vi "io_set_VISA_timeout.vi"(8 "error in":errorcluster caption="error in (no error)", 10 "VISA Timeout":u32=5000, 11 "VISA resource name":refnum<visa-resource-name>) -> (0 "error out":errorcluster, 2 "Old VISA Timeout":u32, 3 "VISA resource name out":refnum<visa-resource-name>)   [LabVIEW 2022 SP3, in "hmp4000_rsidr_core.lvlib"]
uses:
  hmp4000_rsidr_core.lvlib
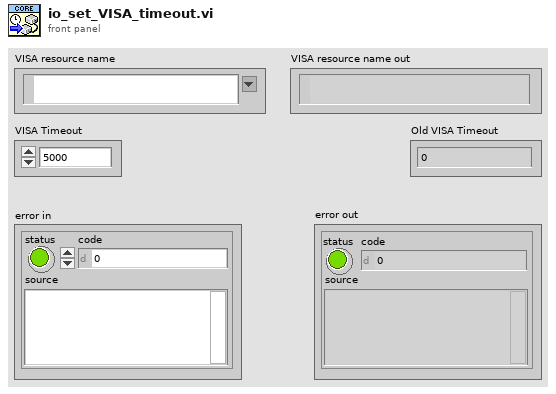
[diagram p1: front panel]
types:
  T1 = typedef "hmp4000_rsidr_core.lvlib/type_Session_Data.ctl" = cluster{"IDN string":string, "Instrument FW":string, "Instr type":string, "Instr type for err. msg.":string, "Installed Options":string[], "Ignore Error Messages":string, "Logging params":variant, "OPC Timeout":i32, "VISA Timeout":i32, "STB Poll VISA Timeout":i32, "Additional Flags":i32, "Wait Before Read":i32, "Wait Before Write":i32, "Option String Flags":i32, "IO Segment Size":i64, "VISA Access Mode":T2, "Interface Type":T3, "OPC Wait Mode":T4, "Bin Float Number  Format":T5, "Bin Integer Number Format":T6, "Simulate":bool, "VXIcapable":bool, "Duplicate Session":bool, "Add LF to Write":bool, "Logging":bool, "Fast Sweep":bool, "Query Instrument Status":bool, "Check Range":bool, "Check Options":bool}
  T2 = typedef "hmp4000_rsidr_core.lvlib/type_VisaAccessMode.ctl" = u16
  T3 = typedef "hmp4000_rsidr_core.lvlib/type_InterfaceType.ctl" = enum16{"Unknown", "GPIB", "VXI", "GPIB_VXI", "ASRL", "PXI", "TCPIP", "USB", "SOCKET"}
  T4 = typedef "hmp4000_rsidr_core.lvlib/type_OPC_Wait_Mode.ctl" = enum16{"STBpolling", "STBpollingSlow", "STBpollingSuperSlow", "ServiceRequest", "OPCquery"}
  T5 = typedef "hmp4000_rsidr_core.lvlib/type_Binary_Float_Number_Format.ctl" = enum16{"Float_4_Bytes_Swapped", "Float_4_Bytes", "Double_8_Bytes_Swapped", "Double_8_Bytes"}
  T6 = typedef "hmp4000_rsidr_core.lvlib/type_Binary_Integer_Number_Format.ctl" = enum16{"Int32_4_Bytes_Swapped", "Int32_4 Bytes", "Int16_2_Bytes_Swapped", "Int16_2_Bytes"}
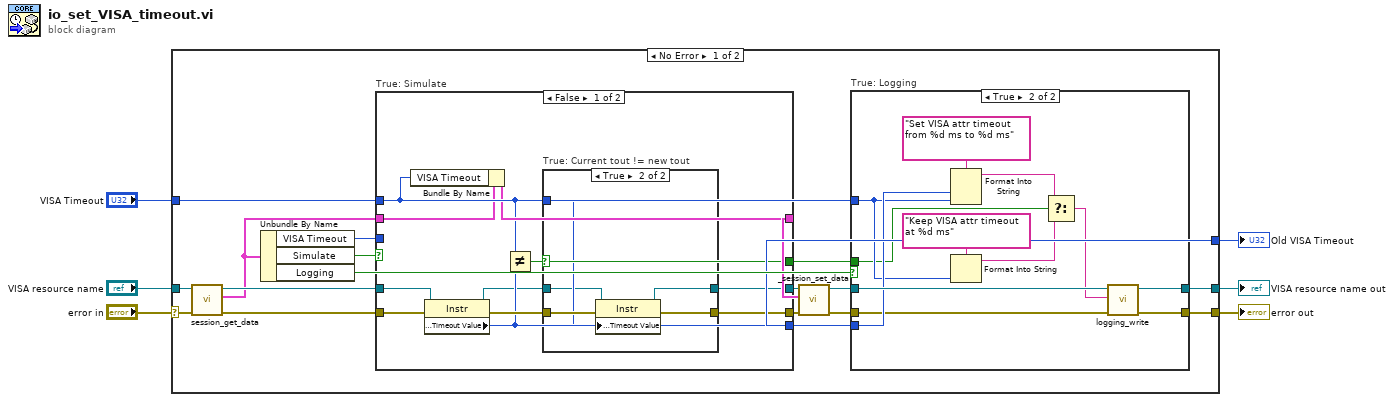
[diagram p0: block diagram]
diagram:
  n1 = case shown="No Error" "error in" {
    selector: "error in" -> [w24 w62]
    tunnel: [w18 w62] -> w4
    tunnel: "VISA resource name" -> [w23 w61]
    tunnel: [w15 w61] -> w3
    tunnel: [w17 w63] -> w2
    tunnel: "VISA Timeout" -> [w19 w63]
    frame No Error {
      n2 = call "session_get_data.vi"("error in"=w24, "VISA resource name"=w23) -> ("error out"=w16:errorcluster, "Session User Data out"=w8:T1, "VISA resource name out"=w22:refnum<visa-resource-name>)  [unwired: 6 in, 1 out]
      n3 = Unbundle By Name(w8) -> ("VISA Timeout"=w9:i32, "Simulate"=w21:bool, "Logging"=w20:bool)
      n4 = case "True: Simulate" shown="False" w21 {
        tunnel: w16 -> [w49 w60]
        tunnel: [w47 w60] -> w13
        tunnel: [w46 w59] -> w12
        tunnel: w22 -> [w45 w59]
        tunnel: [w44 w58] -> w17
        tunnel: w19 -> [w39 _]
        tunnel: [w43 _] -> w14
        tunnel: w9 -> [_ w58]
        tunnel: w8 -> [w42 w57]
        tunnel: [w41 w57] -> w7
        frame False {
          n5 = Bundle By Name(cluster=w42, "VISA Timeout"=w39) -> (w41:T1)
          n6 = property on="Property Node" class="Instr"(reference=w45, error in=w49) -> (reference out=w40:refnum<visa-resource-name>, error out=w48:errorcluster, "General Settings:Timeout Value"=w44:u32)
          n7 = Not Equal?(x=w39, y=w44) -> (x != y?=w43:bool)
          n8 = case "True: Current tout != new tout" shown="True" w43 {
            tunnel: w48 -> [w50 w56]
            tunnel: [w50 w55] -> w47
            tunnel: [w51 w53] -> w46
            tunnel: w40 -> [w51 w52]
            tunnel: w39 -> [_ w54]
            frame False {
            }
            frame True {
              n9 = property on="Property Node" class="Instr"(reference=w52, error in=w56, "General Settings:Timeout Value"=w54) -> (reference out=w53:refnum<visa-resource-name>, error out=w55:errorcluster)
            }
          }
        }
        frame True {
        }
      }
      n10 = call "_session_set_data.vi"("error in"=w13, "Session User Data in"=w7, "VISA resource name"=w12) -> ("error out"=w11:errorcluster, "VISA resource name out"=w10:refnum<visa-resource-name>)  [unwired: 7 in]
      n11 = case "True: Logging" shown="True" w20 {
        tunnel: w19 -> [_ w32]
        tunnel: w10 -> [w25 w38]
        tunnel: w11 -> [w26 w35]
        tunnel: [w26 w34] -> w18
        tunnel: w17 -> [_ w36]
        tunnel: [w25 w33] -> w15
        tunnel: w14 -> [_ w27]
        frame False {
        }
        frame True {
          n12 = Format Into String(format string="Set VISA attr timeout from %d ms to %d ms", w36, w32) -> (resulting string=w30:string)  [unwired: 2 in, 1 out]
          n13 = Format Into String(format string="Keep VISA attr timeout at %d ms", w32) -> (resulting string=w29:string)  [unwired: 2 in, 1 out]
          n14 = Select(t=w30, s=w27, f=w29) -> (s? t:f=w28:string)
          n15 = call "logging_write.vi"("error in"=w35, "String to write"=w28, "VISA resource name"=w38) -> ("error out"=w34:errorcluster, "VISA resource name out"=w33:refnum<visa-resource-name>)  [unwired: 7 in]
        }
      }
    }
    frame Error {
    }
  }
  "VISA resource name out" <- w3
  "error out" <- w4
  "Old VISA Timeout" <- w2
